vi "Auton-MoveToTote.vi"() -> (2 "Task Complete":bool)   [LabVIEW 2014]
uses:
  <vilib>/Rock Robotics/WPI/RobotDrive/WPI_RobotDriveGetSetRefNum.vi
  Robot Global Data.vi
  <vilib>/Rock Robotics/WPI/RobotDrive/WPI_RobotDriveArcadeDrive_Standard(NoSaturation).vi
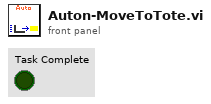
[diagram p1: front panel]
types:
  T1 = typedef "WPI_RobotDriveDevRef.ctl" = cluster{"DevStatus":errorcluster, "Motors[]":T2[], "Square Inputs":bool, "Max Output":dbl}
  T2 = typedef "WPI_MotorControlDeviceRef.ctl" = cluster{"DeviceStatus":errorcluster, "Type":T3, "PWM":cluster{"Controller":T4, "PWM Channel":T5, "DeadBand":T6}, "CAN":cluster{"Device Number":u8, "Control Mode":T7, "Semaphore":T8, "Max Vout":dbl, "TalonSRX Control Mode":T9}, "Invert":bool, "TransformRef":T10, "InvTransformRef":T10}
  T3 = typedef "WPI_MotorControlType.ctl" = enum16{"PWM", "CAN", "CANTalonSRX"}
  T4 = typedef "FPGA_TypedefDigitalModule.ctl" = enum16{"Controller 1"}
  T5 = typedef "FPGA_DIOPWMChannel.ctl" = enum8{"PWM 0", "PWM 1", "PWM 2", "PWM 3", "PWM 4", "PWM 5", "PWM 6", "PWM 7", "PWM 8", "PWM 9", "PWM MXP 0", "PWM MXP 1", "PWM MXP 2", "PWM MXP 3", "PWM MXP 4", "PWM MXP 5", "PWM MXP 6", "PWM MXP 7", "PWM MXP 8", "PWM MXP 9", "Invalid"}
  T6 = typedef "WPI_PWMDeadband.ctl" = cluster{"Name":string, "maxPositivePwm":i32, "minPositivePwm":i32, "centerPwm":i32, "maxNegativePwm":i32, "minNegativePwm":i32, "angularRange":u16}
  T7 = typedef "WPI_CANJaguar_ControlMode.ctl" = enum8{"Percent VBus", "Current", "Speed", "Position", "Voltage"}
  T8 = typedef "Semaphore RefNum" = refnum<k1>
  T9 = typedef "WPI_CANTalonSRX_APIControlMode.ctl" = enum8{"Percent VBus", "Speed", "Position", "Slave", "Unchanged / Invalid"}
  T10 = typedef "WPI_PWMTransform_ConPane.ctl" = refnum<vi>
  T11 = cluster{"Area":dbl, "Number of Holes":dbl, "Bounding Rect":cluster{"Left":dbl, "Top":dbl, "Right":dbl, "Bottom":dbl}, "Center of Mass":cluster{"X":dbl, "Y":dbl}, "Orientation":dbl, "Dimensions":cluster{"Width":dbl, "Height":dbl}}
  T12 = typedef "WPI_DigitalInputDevRef.ctl" = cluster{"DevStatus":errorcluster, "DIO Channel":T13, "Controller":T4}
  T13 = typedef "FPGA_DIOChannel.ctl" = enum8{"DIO 0", "DIO 1", "DIO 2", "DIO 3", "DIO 4", "DIO 5", "DIO 6", "DIO 7", "DIO 8", "DIO 9", "DIO MXP 0", "DIO MXP 1", "DIO MXP 2", "DIO MXP 3", "DIO MXP 4", "DIO MXP 5", "DIO MXP 6", "DIO MXP 7", "DIO MXP 8", "DIO MXP 9", "DIO MXP 10", "DIO MXP 11", "DIO MXP 12", "DIO MXP 13", "DIO MXP 14", "DIO MXP 15", "Invalid"}
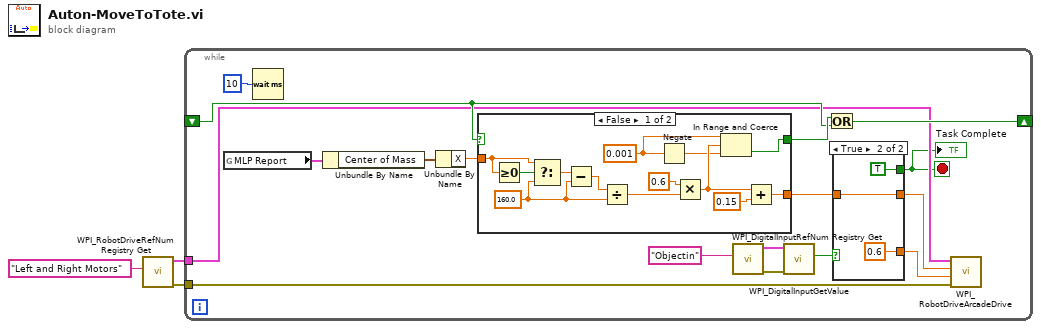
[diagram p0: block diagram]
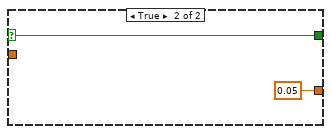
[diagram p2: hidden frame]
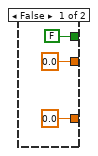
[diagram p3: hidden frame]
diagram:
  n1 = call <vilib>:"WPI_RobotDriveRefNum Registry Get.vi"("refnum name"="Left and Right Motors") -> ("error out"=w1:errorcluster, "RobotDriveDevRef"=w2:T1)  [unwired: 9 in]
  n2 = while {
    tunnel: w2 -> [w5]
    tunnel: w1 -> [w10]
    shift-right: [w8] -> _
    shift-left: _ -> [w9]
    stop <- w4 stop-if-true
    n3 = global read "Robot Global Data.vi" "MLP Report"() -> (w7:T11)
    n4 = Wait (ms)(milliseconds to wait=u32 10) -> ()  [unwired: 1 out]
    n5 = Unbundle By Name(w7) -> ("Center of Mass"=w6:cluster{"X":dbl, "Y":dbl})
    n6 = Unbundle By Name(w6) -> ("X"=w17:dbl)
    n7 = case shown="False" w9 {
      selector: w9 -> [_ w35]
      tunnel: w17 -> [w21 _]
      tunnel: [w26 0.05] -> w16
      tunnel: [w22 w35] -> w11
      frame False {
        w23 = 0.001
        w31 = 160.0 ("f")
        n8 = Greater Or Equal To 0?(x=w21) -> (x >= 0?=w33:bool)
        n9 = Select(t=w21, s=w33, f=w31) -> (s? t:f=w30:dbl)
        n10 = Subtract(x=w30, y=w31) -> (x-y=w32:dbl)
        n11 = Divide(x=w32, y=w31) -> (x/y=w29:dbl)
        n12 = Negate(x=w23) -> (-x=w24:dbl)
        n13 = Multiply(x=0.6, y=w29) -> (x*y=w25:dbl)
        n14 = In Range and Coerce(upper limit=w23, x=w25, lower limit=w24) -> (In Range?=w22:bool)  [unwired: 1 out]
        n15 = Add(x=w25, y=0.15) -> (x+y=w26:dbl)
      }
      frame True {
      }
    }
    n16 = call <vilib>:"WPI_DigitalInputRefNum Registry Get.vi"("refnum name"="Objectin") -> ("error out"=w15:errorcluster, "DigitalInputDevRef"=w12:T12)  [unwired: 9 in]
    n17 = call <vilib>:"WPI_DigitalInputGetValue.vi"("error in (no error)"=w15, "DigitalInputDevRef"=w12) -> ("Value"=w14:bool)  [unwired: 7 in, 2 out]
    n18 = Or(x=w11, y=w9) -> (x .or. y?=w8:bool)
    n19 = case shown="True" w14 {
      tunnel: [0.0 ("X axis value") 0.6 ("X axis value")] -> w20
      tunnel: [0.0 ("X axis value") w41] -> w19
      tunnel: w16 -> [_ w41]
      tunnel: [FALSE TRUE] -> w4
      frame False {
      }
      frame True {
      }
    }
    "Task Complete" <- w4
    n20 = call-poly <vilib>:"WPI_RobotDriveArcadeDrive.vi"("error in (no error)"=w10, "Y axis value"=w20, "X axis value"=w19, "RobotDriveDevRef"=w5) -> ()  [unwired: 8 out]
  }
